vi "Build One Term Numeric Functions - Signed Types.vi"(11 "Function Name":string) -> ()   [LabVIEW 2021]
uses:
  <vilib>/numeric/LVNumericRepresentation.ctl
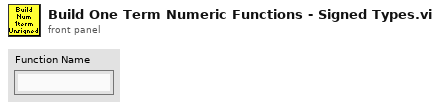
[diagram p1: front panel]
types:
  T1 = typedef "LVNumericRepresentation.ctl" = enum32{"Extended Precision", "Double Precision", "Single Precision", "Long", "Word", "Byte", "Unsigned Long", "Unsigned Word", "Unsigned Byte", "Complex Extended", "Complex Double", "Complex Single", "Quad", "Unsigned Quad", "Fixed-Point"}
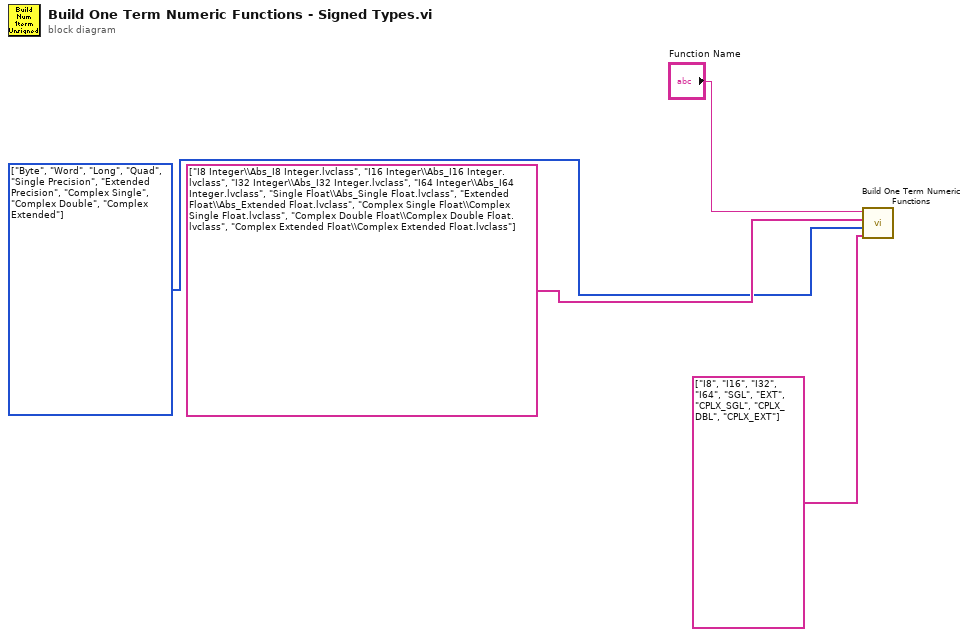
[diagram p0: block diagram]
diagram:
  w3 = T1[] [enum."Byte", enum."Word", enum."Long", enum."Quad", enum."Single Precision", enum."Extended Precision", enum."Complex Single", enum."Complex Double", enum."Complex Extended"] items=["Extended Precision", "Double Precision", "Single Precision", "Long", "Word", "Byte", "Unsigned Long", "Unsigned Word", "Unsigned Byte", "Complex Extended", "Complex Double", "Complex Single", "Quad", "Unsigned Quad", "Fixed-Point"] ("Representation")
  n1 = call "Build One Term Numeric Functions.vi"("Names"=string[] ["I8", "I16", "I32", "I64", "SGL", "EXT", "CPLX_SGL", "CPLX_DBL", "CPLX_EXT"], "Representation"=w3, "Abstract Type Locations"=string[] ["I8 Integer\\Abs_I8 Integer.lvclass", "I16 Integer\\Abs_I16 Integer.lvclass", "I32 Integer\\Abs_I32 Integer.lvclass", "I64 Integer\\Abs_I64 Integer.lvclass", "Single Float\\Abs_Single Float.lvclass", "Extended Float\\Abs_Extended Float.lvclass", "Complex Single Float\\Complex Single Float.lvclass", "Complex Double Float\\Complex Double Float.lvclass", "Complex Extended Float\\Complex Extended Float.lvclass"], "Comparison Name"="Function Name") -> ()  [unwired: 8 in]
